vi "Camera_ID.vi"(8 "error in":errorcluster) -> (0 "error out":errorcluster, 1 "Camera1":string, 3 "Camera2":string)   [LabVIEW 2020]
uses:
  <vilib>/vision/driver/NI_Vision_Acquisition_Software.lvlib
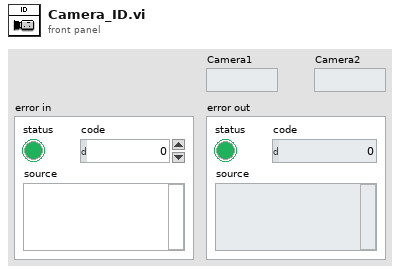
[diagram p1: front panel]
types:
  T1 = cluster{"Type":u32, "Version":u32, "Flags":u32, "SerialNumberHigh":u32, "SerialNumberLow":u32, "BusType":u32, "InterfaceName":string, "VendorName":string, "ModelName":string, "CameraFileName":string, "CameraAttributeURL":string}[]
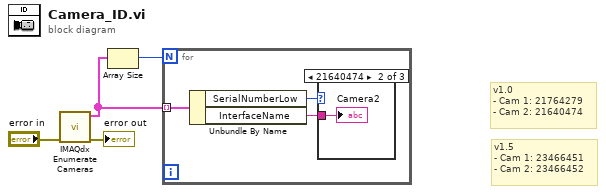
[diagram p0: block diagram]
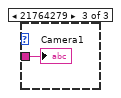
[diagram p3: hidden frame]
diagram:
  # "v1.5\n- Cam 1: 23466451 \n- Cam 2: 23466452"
  # "v1.0\n- Cam 1: 21764279 \n- Cam 2: 21640474"
  n1 = call <vilib>:"IMAQdx Enumerate Cameras.vi"("error in"="error in") -> ("error out"=→"error out":errorcluster, "Camera Information Array"=w3:T1)  [unwired: 9 in]
  n2 = Array Size(array=w3) -> (size(s)=w4:i32)
  n3 = for {
    N: w4 -> [_]
    tunnel: w3 -> [w7] mode=indexing
    n4 = Unbundle By Name(w7) -> ("SerialNumberLow"=w5:u32, "InterfaceName"=w6:string)
    n5 = case shown="21640474" w5 {
      tunnel: w6 -> [_ w8 w9]
      frame 0, Default {
      }
      frame 21640474 {
        "Camera2" <- w8
      }
      frame 21764279 {
        "Camera1" <- w9
      }
    }
  }
